vi "Remove Sensor.vi"(8 "error in (no error)":errorcluster, 10 "Name":string, 11 "Sensor List Class in":refnum<class "Sensor List Class.lvclass">) -> (0 "error out":errorcluster, 3 "Sensor List Class out":refnum<class "Sensor List Class.lvclass">)   [LabVIEW 2013, in "Sensor List Class.lvclass"]
uses:
  Sensor List Class.lvclass
  Sensor List Class.lvclass/Sensor List Class.ctl
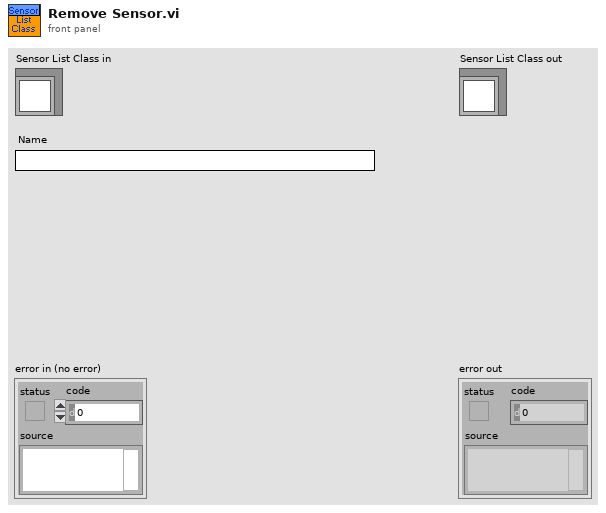
[diagram p1: front panel]
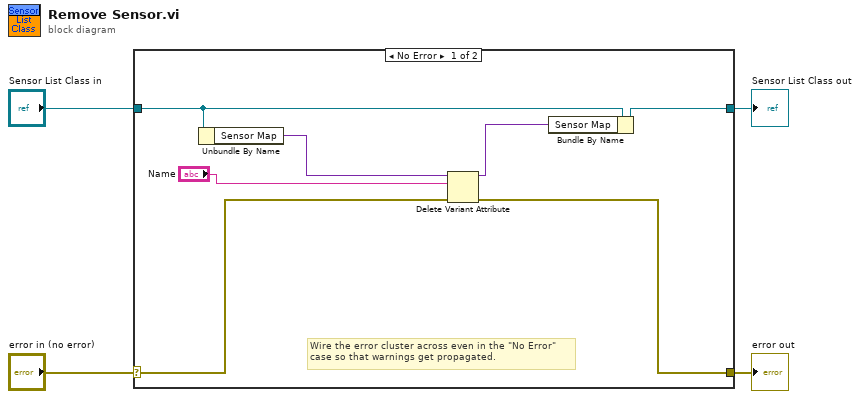
[diagram p0: block diagram]
diagram:
  n1 = case shown="No Error" "error in (no error)" {
    selector: "error in (no error)" -> [w6 w13]
    tunnel: [w5 w13] -> w3
    tunnel: [w10 w12] -> w1
    tunnel: "Sensor List Class in" -> [w9 w12]
    frame No Error {
      # "Wire the error cluster across even in the \"No Error\"\ncase so that warnings get propagated."
      n2 = Unbundle By Name(w9) -> ("Sensor Map"=w8:variant)
      n3 = Delete Variant Attribute(4:w6, 6:"Name", 7:w8) -> (0:w5:errorcluster, 3:w7:variant)  [unwired: 1 out]
      n4 = Bundle By Name(cluster=w9, "Sensor Map"=w7) -> (w10:refnum<class "Sensor List Class.lvclass">)
    }
    frame Error {
    }
  }
  "error out" <- w3
  "Sensor List Class out" <- w1
